vi "Configure Trigger.vi"(8 "error in (no error)":errorcluster, 10 "Trigger Source(0:Immediate)":u16(ring) items=["Immediate", "External", "BUS"], 11 "VISA resource name":refnum<visa-resource-name>) -> (0 "error out":errorcluster, 3 "VISA resource name out":refnum<visa-resource-name>)   [LabVIEW 2021, in "Keithley 2200 Series.lvlib"]
doc: "Configure the trigger settings on the instrument."
uses:
  <instrlib>/Keithley 2200 Series/Keithley 2200 Series.lvlib
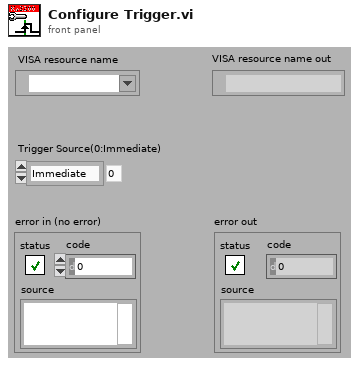
[diagram p1: front panel]
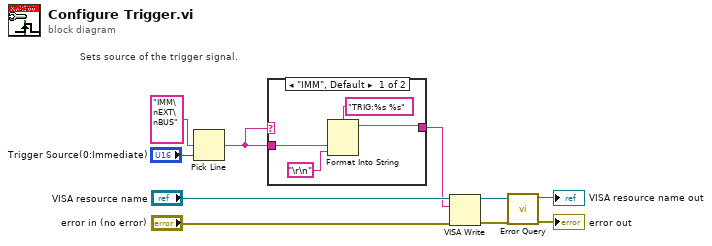
[diagram p0: block diagram]
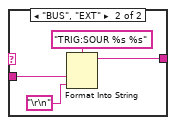
[diagram p2: hidden frame]
diagram:
  # "Sets source of the trigger signal."
  n1 = Pick Line(multi-line string="IMM\nEXT\nBUS", line index="Trigger Source(0:Immediate)") -> (output string=w1:string)  [unwired: 1 out]
  n2 = case shown="\"IMM\", Default" w1 {
    tunnel: w1 -> [w12 w17]
    tunnel: [w11 w15] -> w2
    frame "IMM", Default {
      n3 = Format Into String(format string="TRIG:%s %s", w12, "\r\n" ("End of Line Constant")) -> (resulting string=w11:string)  [unwired: 2 in, 1 out]
    }
    frame "BUS", "EXT" {
      n4 = Format Into String(format string="TRIG:SOUR %s %s", w17, "\r\n" ("End of Line Constant")) -> (resulting string=w15:string)  [unwired: 2 in, 1 out]
    }
  }
  n5 = VISA Write(VISA resource name="VISA resource name", write buffer=w2, error in (no error)="error in (no error)") -> (VISA resource name out=w6:refnum<visa-resource-name>, error out=w5:errorcluster)  [unwired: 1 out]
  n6 = call <instrlib>:"Error Query.vi"("error in (no error)"=w5, "VISA resource name"=w6) -> ("error out"=→"error out":errorcluster, "VISA resource name out"=→"VISA resource name out":refnum<visa-resource-name>)  [unwired: 8 out]
